vi "Reshape.vi"(6 "feature/ch":i32, 9 "EEG_Channel_Num":i32, 10 "all rows":dbl[][](array[numeric]), 11 "Trial_number":dbl) -> (3 "Array":dbl[][](array[numeric]))   [LabVIEW 2013]
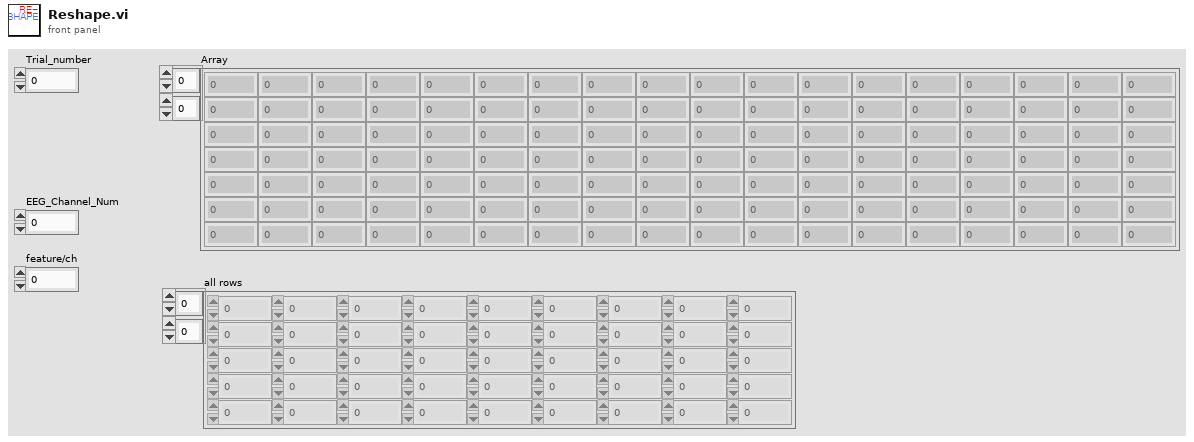
[diagram p1: front panel]
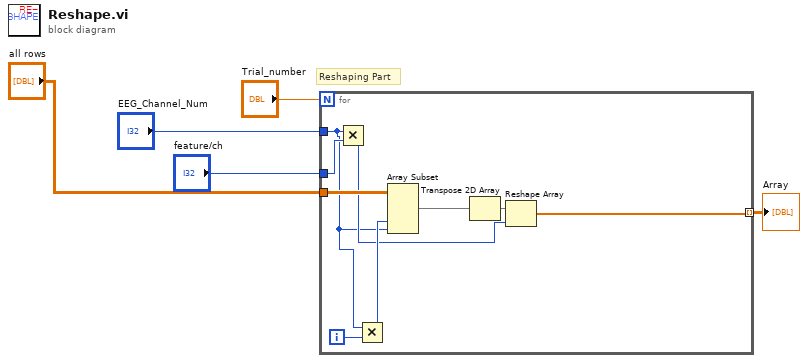
[diagram p0: block diagram]
diagram:
  # "Reshaping Part"
  n1 = for {
    N: "Trial_number" -> [_]
    tunnel: "EEG_Channel_Num" -> [w8]
    tunnel: "all rows" -> [w14]
    tunnel: "feature/ch" -> [w12]
    tunnel: [w9] -> w5 mode=indexing
    i -> [w13]
    n2 = Multiply(x=w8, y=w12) -> (x*y=w10:i32)
    n3 = Multiply(x=w8, y=w13) -> (x*y=w11:i32)
    n4 = Array Subset(array=w14, index (col)=w11, length (col)=w8) -> (w7:dbl[][])  [unwired: 2 in]
    n5 = Transpose 2D Array(2D array=w7) -> (transposed array=w6:dbl[][])
    n6 = Reshape Array(w6, w10) -> (w9:dbl[])
  }
  "Array" <- w5
